vi "TAI Time to LabVIEW Time.vi"(5 "TAI Time (ns)":i64) -> (2 "LabVIEW Time (s)":timestamp)   [LabVIEW 2021, in "Time_CIF_U.lvlib"]
doc: "Convert TAI time into LabVIEW time by changing the epoch. TAI time is used as the basis of UTC and is GPS time. It is UTC without leap seconds."
uses:
  Time_CIF_U.lvlib
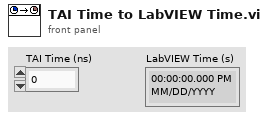
[diagram p1: front panel]
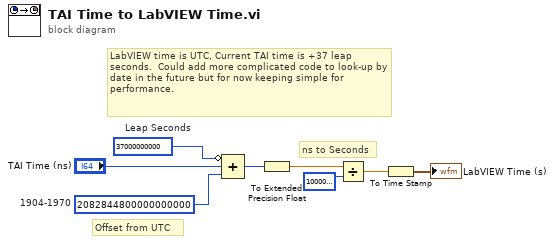
[diagram p0: block diagram]
diagram:
  w4 = i64 37000000000  # Leap Seconds
  w2 = i64 2082844800000000000  # 1904-1970
  # "LabVIEW time is UTC, Current TAI time is +37 leap seconds.  Could add more complicated code to look-up by date in the future but for now keeping simple for performance."
  # "Offset from UTC"
  # "ns to Seconds"
  n1 = Compound Arithmetic op=ADD(invert w4, "TAI Time (ns)", w2) -> (w1:i64)
  n2 = To Extended Precision Float(1:w1) -> (0:w5:ext)
  n3 = Divide(x=w5, y=u64 1000000000) -> (x/y=w8:ext)
  n4 = To Time Stamp(1:w8) -> (0:→"LabVIEW Time (s)":timestamp)
